vi "return error.vi"(8 "error in (no error)":errorcluster, 11 "return code":i32) -> (0 "error out":errorcluster)   [LabVIEW 2015]
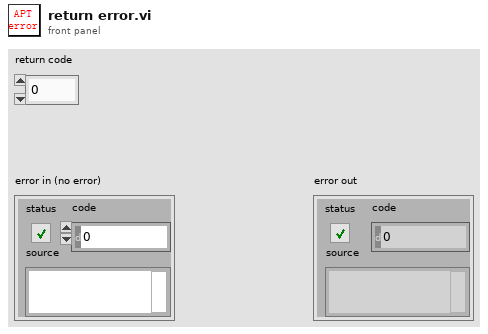
[diagram p1: front panel]
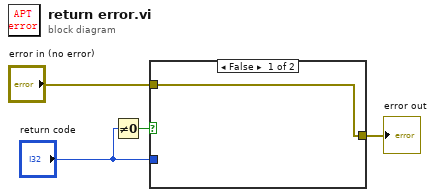
[diagram p0: block diagram]
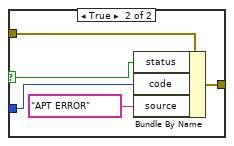
[diagram p2: hidden frame]
diagram:
  n1 = Not Equal To 0?(x="return code") -> (x != 0?=w4:bool)
  n2 = case shown="False" w4 {
    selector: w4 -> [_ w9]
    tunnel: "error in (no error)" -> [w5 w10]
    tunnel: "return code" -> [_ w8]
    tunnel: [w5 w6] -> w1
    frame False {
    }
    frame True {
      n3 = Bundle By Name(cluster=w10, "status"=w9, "code"=w8, "source"="APT ERROR") -> (w6:errorcluster)
    }
  }
  "error out" <- w1
